vi "2.Réservoir.vi"() -> ()   [LabVIEW 2018]
panel:
  in  "Consigne":i16(slide) min=0 max=1000 scale=0.0..1000.0
  in  "Débit":dbl(slide) scale=0.0..10.0
  in  "stop":bool
  in  "Conisgne":dbl
  out "Tank":i16(slide) scale=0.0..1000.0
  # "1/s"
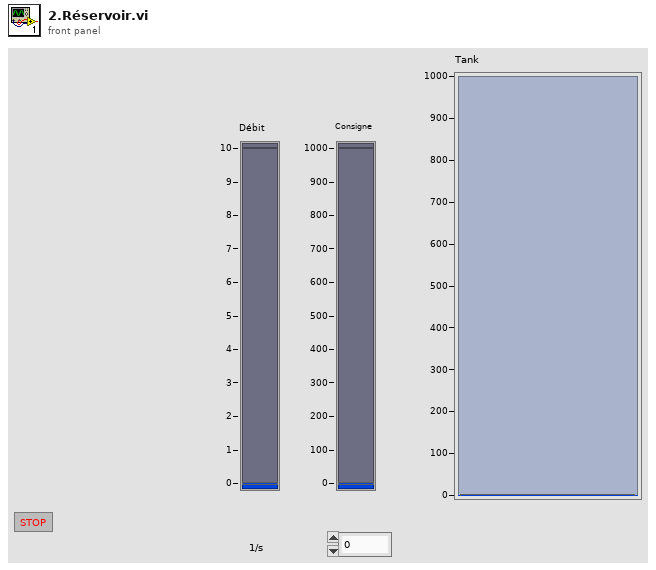
[diagram p1: front panel]
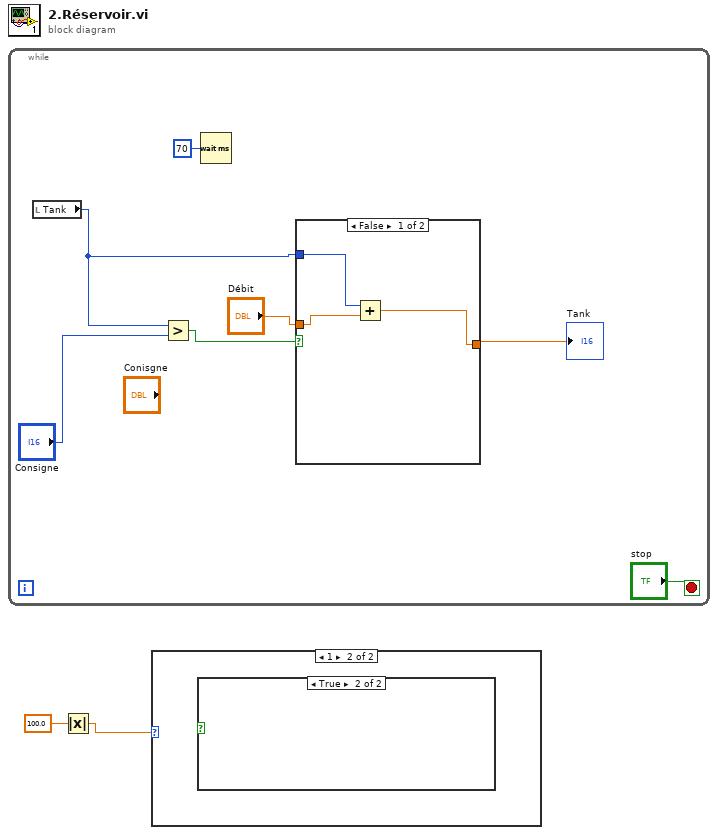
[diagram p0: block diagram]
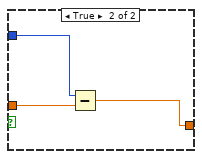
[diagram p4: hidden frame]
diagram:
  n1 = while {
    stop <- "stop" stop-if-true
    n2 = local read "Tank"() -> (w8:i16)
    n3 = Greater?(x=w8, y="Consigne") -> (0:w9:bool)
    n4 = Wait (ms)(milliseconds to wait=u32 70) -> ()  [unwired: 1 out]
    n5 = case shown="False" w9 {
      tunnel: w8 -> [w12 w15]
      tunnel: [w11 w14] -> w7
      tunnel: "Débit" -> [w10 w13]
      frame False {
        n6 = Add(x=w12, y=w10) -> (x+y=w11:dbl)
      }
      frame True {
        n7 = Subtract(x=w15, y=w13) -> (x-y=w14:dbl)
      }
    }
    "Tank" <- w7
  }
  n8 = Absolute Value(x=100.0) -> (abs(x)=w1:dbl)
  n9 = case shown="1" w1 {
    frame 0, Default {
    }
    frame 1 {
      n10 = case shown="True" {
        selector: _ -> [_ _]
        frame False {
        }
        frame True {
        }
      }
    }
  }
